vi "Read Pots.vi"() -> (0 "Pot Write Cluster":T1, 2 "Right Pot":dbl, 3 "Left Pot":dbl, 4 "Unzeroed Right Pot":dbl, 6 "Unzeroed Left Pot":dbl)   [LabVIEW 2014]
uses:
  Pot Data.ctl
  Robot Global Data.vi
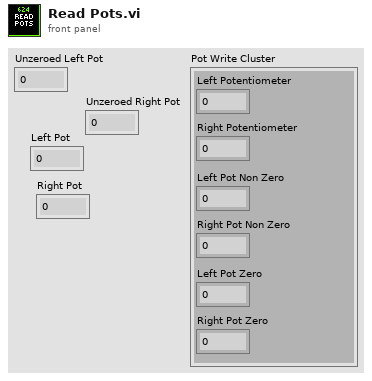
[diagram p1: front panel]
types:
  T1 = typedef "Pot Data.ctl" = cluster{"Left Pot Zero":dbl, "Right Pot Zero":dbl, "Left Potentiometer":dbl, "Right Potentiometer":dbl, "Left Pot Non Zero":dbl, "Right Pot Non Zero":dbl}
  T2 = typedef "Dashboard Control Data.ctl" = cluster{"Cam Exposure":dbl, "Go to angle":dbl, "Steer PID Gains":cluster{"proportional gain (Kc)":dbl, "integral time (Ti, min)":dbl, "derivative time (Td, min)":dbl}, "Steer PID output Range":cluster{"output high":dbl, "output low":dbl}, "Pressure m \nValue":dbl, "Pressure b \nValue":dbl, "Strafe Timer\nWait":dbl, "Roller Command Cluster ":T3, "Elevator":T4, "Strafe Correct min X":dbl, "IMU Enable":bool, "Encoder Control":T6}
  T3 = typedef "Roller Control.ctl" = cluster{"Left Roller Speed":dbl, "Right Roller Speed":dbl, "Left Roller Speed Back":dbl, "Right Roller Speed Back":dbl, "Roller Align Decide Limit":u32, "Left Roller Speed Unload":dbl, "Right Roller Speed Unload":dbl, "Ping Dist Difference":dbl, "Ping In Dist":dbl, "Right Pot 0":dbl, "Pot Threshold":dbl, "Left Pot 0":dbl, "Manual 0s?":bool, "Right Pot Scale":dbl, "Left Pot Scale":dbl, "0 wait time":i32, "Reset?":bool}
  T4 = typedef "Elevator DB Control.ctl" = cluster{"PID Output Range":cluster{"output high":dbl, "output low":dbl}, "PID gains":cluster{"proportional gain (Kc)":dbl, "integral time (Ti, min)":dbl, "derivative time (Td, min)":dbl}, "Height Tolerance":dbl, " Encoder Constant":dbl, "Safe Mode Max Speed":dbl, "Eject Time":dbl, "Encoder Filter?":bool, "Zeroing Speed":dbl, "Presets":T5}
  T5 = typedef "Elevator Presets.ctl" = cluster{"Hold Tote":dbl, "Hold Trashcan":dbl, "Pickup 2 w/ Tote":dbl, "Pickup 2 w/ Trashcan":dbl, "Pickup 3 w/ Tote":dbl, "Pickup 3 w/ Trashcan":dbl, "Bottom":dbl, "Pickup 1 w/ Tote":dbl, "Pickup Trashcan":dbl, "Pickup 1 w/ Trashcan":dbl, "Eject":dbl}
  T6 = typedef "Encoder Control.ctl" = cluster{"Left Tick Constant":dbl, "Right Tick Constant":dbl, "Center Tick Constant":dbl, "Reset?":bool}
  T7 = typedef "WPI_PotentiometerDevRef.ctl" = cluster{"DevStatus":errorcluster, "Controller":T8, "Analog Channel":T9, "Invert Output":bool}
  T8 = typedef "FPGA_TypedefAnalogModule.ctl" = enum16{"Controller 1"}
  T9 = typedef "FPGA_AIChannel.ctl" = enum8{"AI 0", "AI 1", "AI 2", "AI 3", "AI MXP 0", "AI MXP 1", "AI MXP 2", "AI MXP 3", "Invalid"}
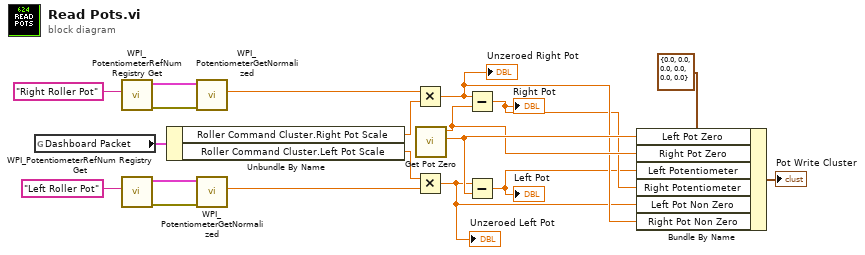
[diagram p0: block diagram]
diagram:
  n1 = global read "Robot Global Data.vi" "Dashboard Packet"() -> (w13:T2)
  n2 = call <vilib>:"WPI_PotentiometerRefNum Registry Get.vi"("refnum name"="Right Roller Pot") -> ("error out"=w19:errorcluster, "PotDevRef"=w18:T7)  [unwired: 9 in]
  n3 = call <vilib>:"WPI_PotentiometerRefNum Registry Get.vi"("refnum name"="Left Roller Pot") -> ("error out"=w16:errorcluster, "PotDevRef"=w17:T7)  [unwired: 9 in]
  n4 = Unbundle By Name(w13) -> ("Roller Command Cluster.Right Pot Scale"=w10:dbl, "Roller Command Cluster.Left Pot Scale"=w9:dbl)
  n5 = call <vilib>:"WPI_PotentiometerGetNormalized.vi"("error in"=w19, "PotDevRef"=w18) -> ("Normalized Value"=w12:dbl)  [unwired: 7 in, 2 out]
  n6 = call <vilib>:"WPI_PotentiometerGetNormalized.vi"("error in"=w16, "PotDevRef"=w17) -> ("Normalized Value"=w11:dbl)  [unwired: 7 in, 2 out]
  n7 = Multiply(x=w12, y=w10) -> (x*y=w5:dbl)
  "Unzeroed Right Pot" <- w5
  n8 = Multiply(x=w9, y=w11) -> (x*y=w4:dbl)
  "Unzeroed Left Pot" <- w4
  n9 = call "Get Pot Zero.vi"() -> ("Left Pot 0"=w7:dbl, "Right Pot 0"=w6:dbl)  [unwired: 10 in]
  n10 = Subtract(x=w5, y=w6) -> (x-y=w3:dbl)
  "Right Pot" <- w3
  n11 = Subtract(x=w4, y=w7) -> (x-y=w2:dbl)
  "Left Pot" <- w2
  n12 = Bundle By Name(cluster=T1 {"Left Pot Zero"=0.0, "Right Pot Zero"=0.0, "Left Potentiometer"=0.0, "Right Potentiometer"=0.0, "Left Pot Non Zero"=0.0, "Right Pot Non Zero"=0.0} ("Potentiometer Cluster"), "Left Pot Zero"=w7, "Right Pot Zero"=w6, "Left Potentiometer"=w2, "Right Potentiometer"=w3, "Left Pot Non Zero"=w4, "Right Pot Non Zero"=w5) -> (→"Pot Write Cluster":T1)
